vi "System Close.vi"(8 "error in (no error)":errorcluster, 10 "Pound":refnum<class "Pound.lvclass">, 11 "Qbus":refnum<class "Qbus.lvclass">) -> (0 "error out":errorcluster)   [LabVIEW 2015, in "Exposure Process.lvlib"]
uses:
  Exposure Process.lvlib
  <vilib>/addons/Qbus/Qbus.lvclass
  <vilib>/NI/Software Watchdog/Pound/Pound.lvclass
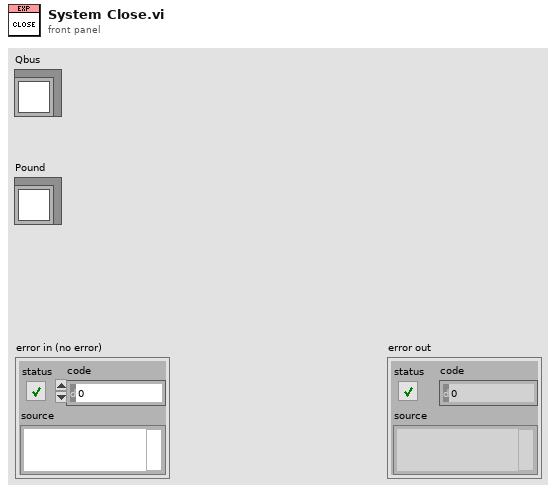
[diagram p1: front panel]
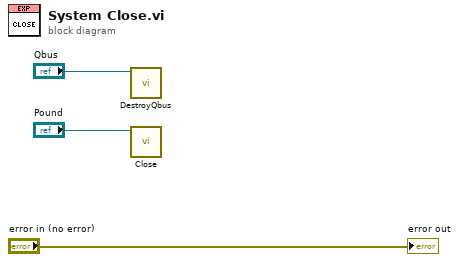
[diagram p0: block diagram]
diagram:
  n1 = call <vilib>:"DestroyQbus.vi"("Qbus"="Qbus") -> ()  [unwired: 10 in, 1 out]
  n2 = call <vilib>:"Close.vi"("Pound"="Pound") -> ()  [unwired: 10 in, 1 out]
  "error out" <- "error in (no error)"
